vi "RangeCheck.vi"(0 "ChromaAcLoad in":refnum<class "ChromaAcLoad.lvclass">, 1 "RangeCheck":T1, 2 "Phase":i32, 3 "error in (no error)":errorcluster) -> (7 "ChromaAcLoad out":refnum<class "ChromaAcLoad.lvclass">, 10 "error out":errorcluster)   [LabVIEW 2018, in "AcPwrPlugins.lvlib" / "ChromaAcLoad.lvclass"]
doc: "This VI checks the value of the instrument settings and returns an error if the value is outside the instrument range."
uses:
  ChromaAcLoad.lvclass
  TypeDefs/RangeCheck.ctl
  <vilib>/Utility/error.llb/Error Cluster From Error Code.vi
  <vilib>/ErrorRing/Error Ring.xnode
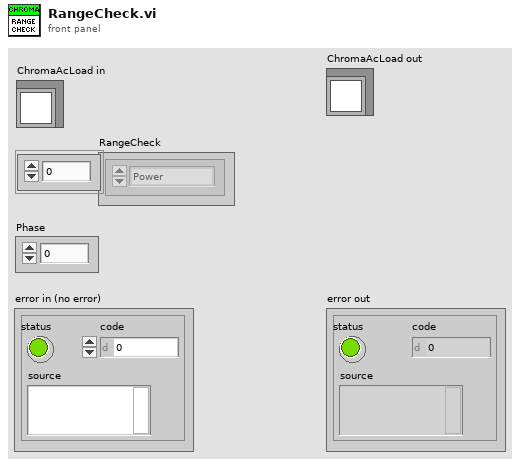
[diagram p1: front panel]
types:
  T1 = typedef "AcPwrPlugins.lvlib/ChromaAcLoad.lvclass/RangeCheck.ctl" = enum16{"Power", "AC Peak Current", "Crest Factor", "Power Factor", "Current Limit", "Current", "RLC Power Factor", "DC Peak Current", "Inrush Peak Current", "RLC Power", "DC Voltage", "AC Voltage", "DC Resistance", "AC Resistance", "Capacitance", "Inductance", "RLC RL", "RLC RS", "Frequency", "Rise Slew Rate", "Fall Slew Rate"}[]
  T2 = typedef "AcPwrPlugins.lvlib/ChromaAcLoad.lvclass/DeviceProperties.ctl" = cluster{"Frequency (Hz)":dbl, "Phases":cluster{"Handle":string, "Name":string, "Phase Select":i32, "option string ":string, "id query (Yes)":bool, "reset device (Yes)":bool, "LC":cluster{"C (uF)":i32, "L (uH)":i32, "RS (Ohm)":dbl, "RL (Ohm)":dbl}, "Load Current (A/Arms)":dbl, "Load Voltage (V/Vrms)":dbl, "Load Power (W)":dbl, "Load Resistance (Ohms)":dbl, "Load Current Peak (A)":dbl, "Load Current Limit (A/Arms)":dbl, "Slew Rate":cluster{"Rise Slew Rate (Units/S)":i32, "Fall Slew Rate (Units/S)":i32}, "Load Short Circuited":bool, "Line Synchronization":bool, "Priority":enum16{"CF Only", "PF Only", "Both (CF)", "Both (PF)"}, "Crest Factor":dbl, "Power Factor":dbl, "Connected":bool, "Voltage Range (V)":dbl[], "Timing":cluster{"TimingOn":enum16{""}, "Hours":u32, "Minutes":u32, "Seconds":dbl, "CutoffVoltage":dbl}}[], "Configuration Mode":enum16{"Constant Voltage (DC)", "Constant Power (DC)", "Constant Power (AC)", "Constant Current (DC)", "Constant Current (AC)", "Constant Resistance (DC)", "Constant Resistance (AC)", "Rectified Mode (DC)", "Inrush (AC)", "RLC CP (AC)", "RLC (AC)"}}[]
  T3 = cluster{"Handle":string, "Name":string, "Phase Select":i32, "option string ":string, "id query (Yes)":bool, "reset device (Yes)":bool, "LC":cluster{"C (uF)":i32, "L (uH)":i32, "RS (Ohm)":dbl, "RL (Ohm)":dbl}, "Load Current (A/Arms)":dbl, "Load Voltage (V/Vrms)":dbl, "Load Power (W)":dbl, "Load Resistance (Ohms)":dbl, "Load Current Peak (A)":dbl, "Load Current Limit (A/Arms)":dbl, "Slew Rate":cluster{"Rise Slew Rate (Units/S)":i32, "Fall Slew Rate (Units/S)":i32}, "Load Short Circuited":bool, "Line Synchronization":bool, "Priority":enum16{"CF Only", "PF Only", "Both (CF)", "Both (PF)"}, "Crest Factor":dbl, "Power Factor":dbl, "Connected":bool, "Voltage Range (V)":dbl[], "Timing":cluster{"TimingOn":enum16{""}, "Hours":u32, "Minutes":u32, "Seconds":dbl, "CutoffVoltage":dbl}}[]
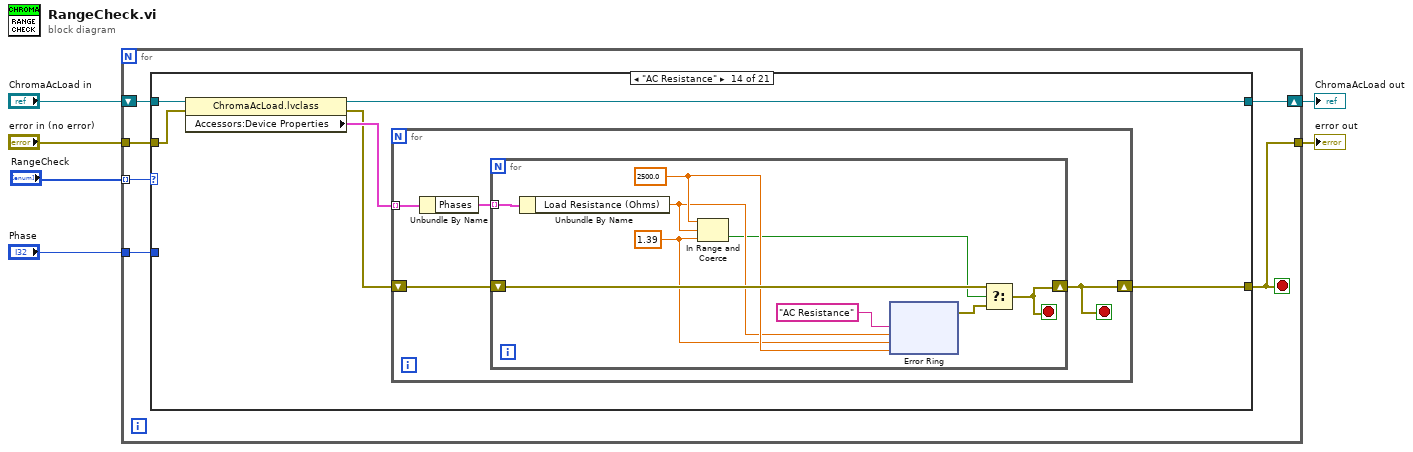
[diagram p0: block diagram]
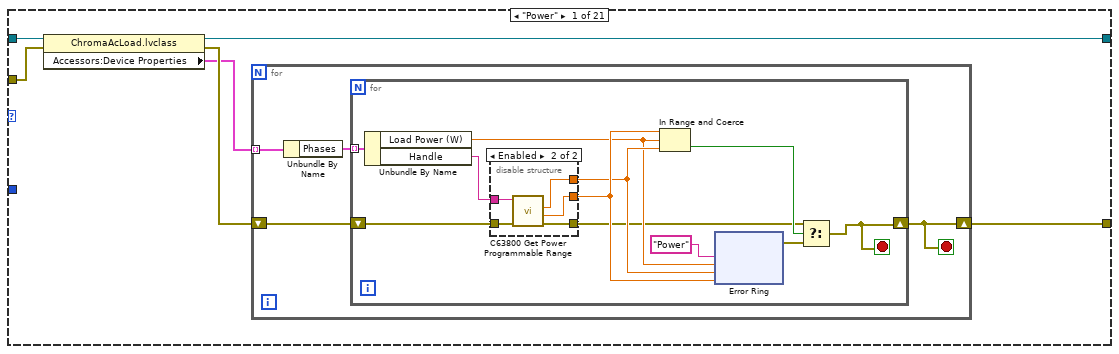
[diagram p2: hidden frame]
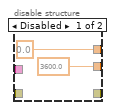
[diagram p3: hidden frame]
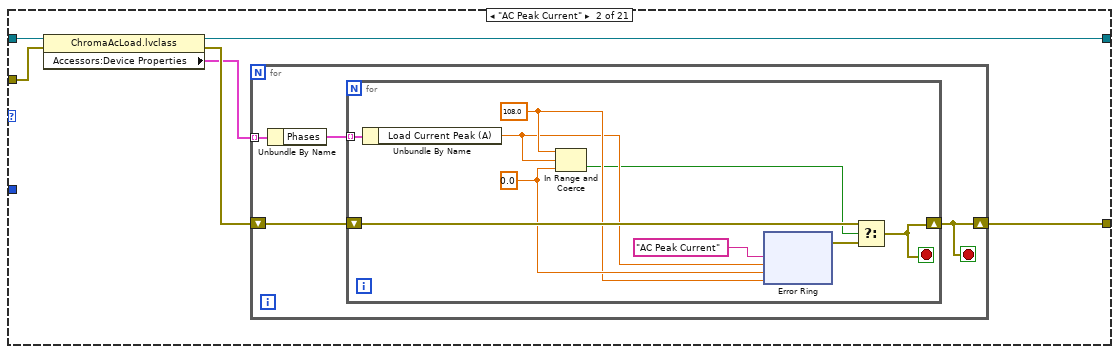
[diagram p4: hidden frame]
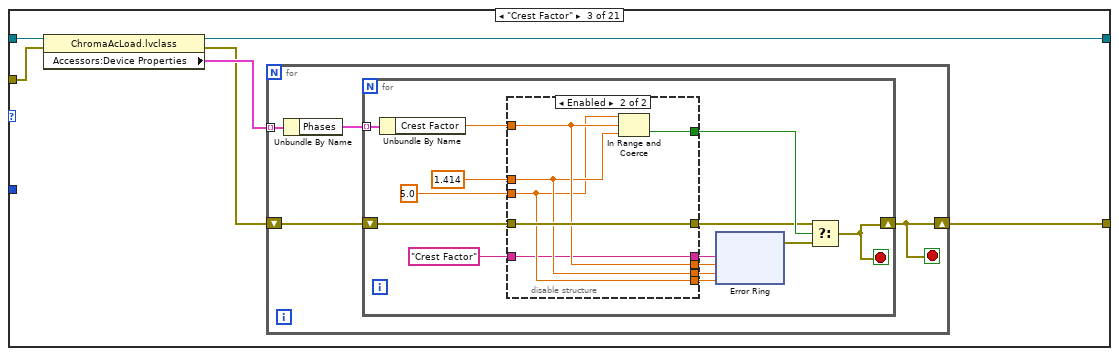
[diagram p5: hidden frame]
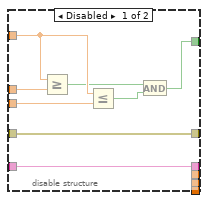
[diagram p6: hidden frame]
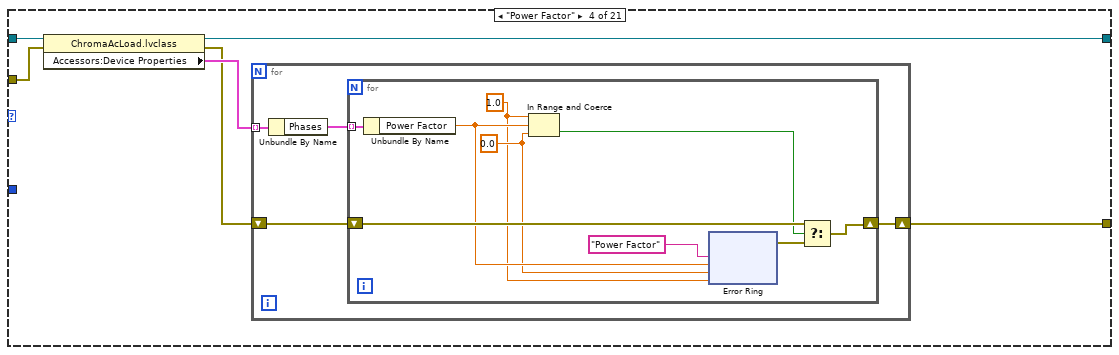
[diagram p7: hidden frame]
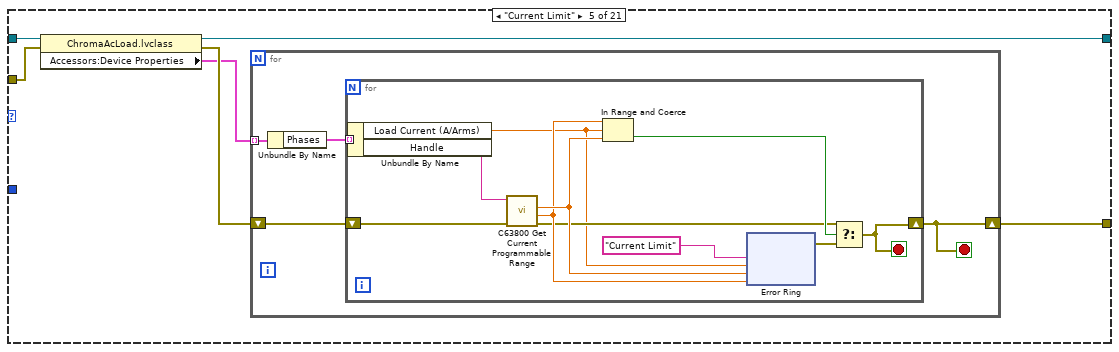
[diagram p8: hidden frame]
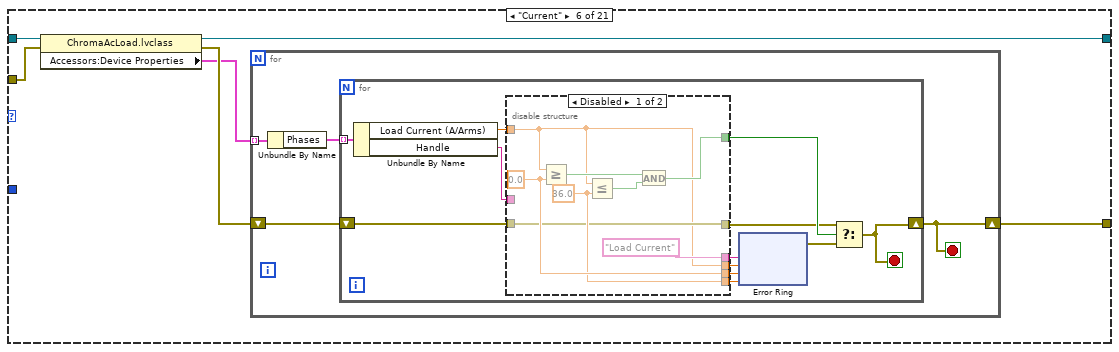
[diagram p9: hidden frame]
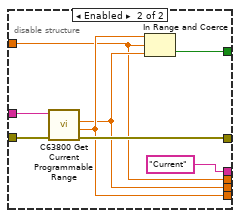
[diagram p10: hidden frame]
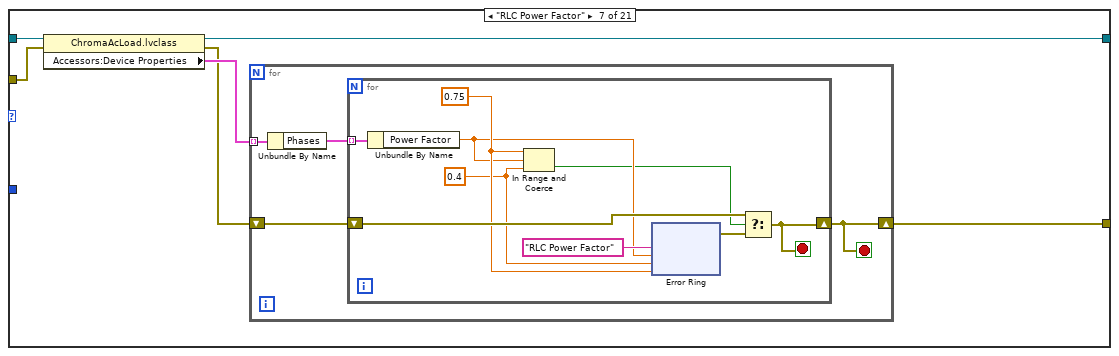
[diagram p11: hidden frame]
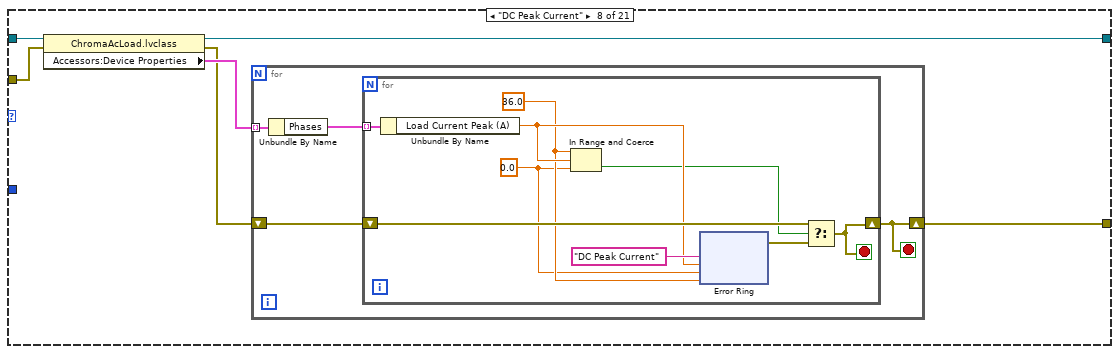
[diagram p12: hidden frame]
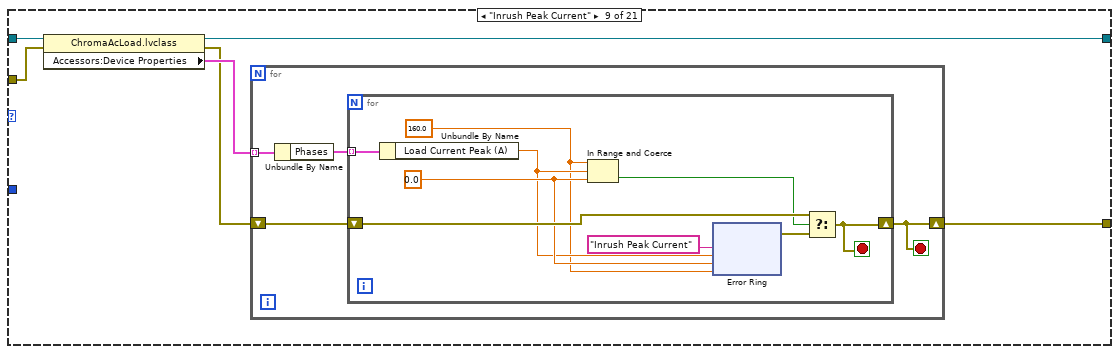
[diagram p13: hidden frame]
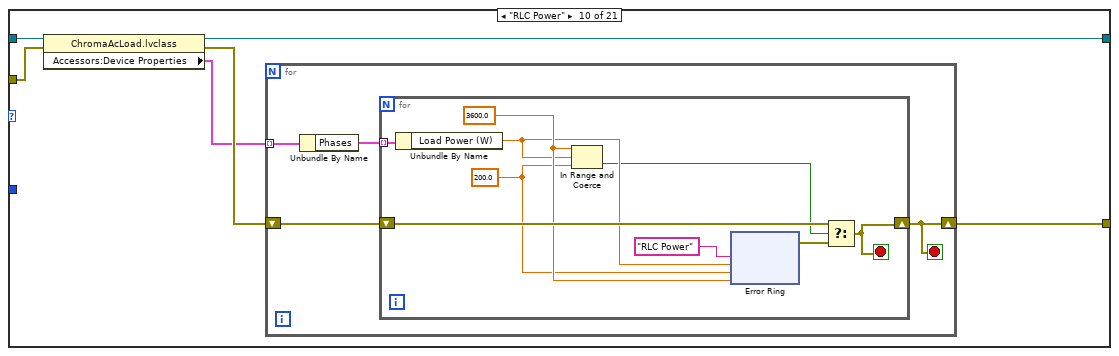
[diagram p14: hidden frame]
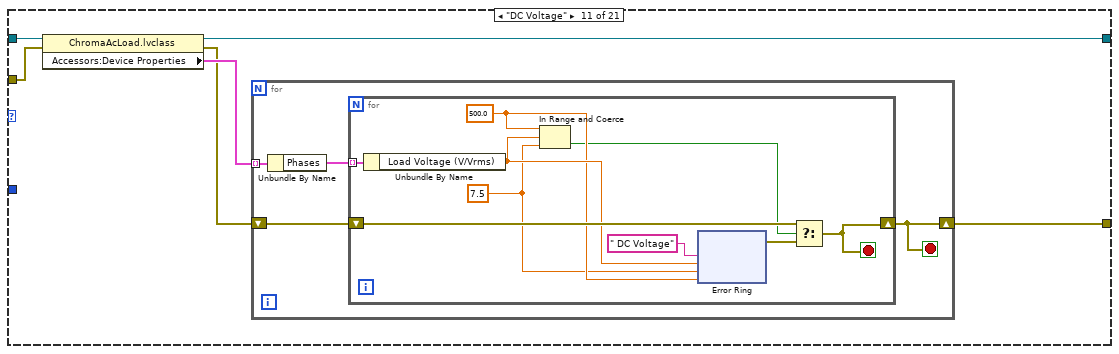
[diagram p15: hidden frame]
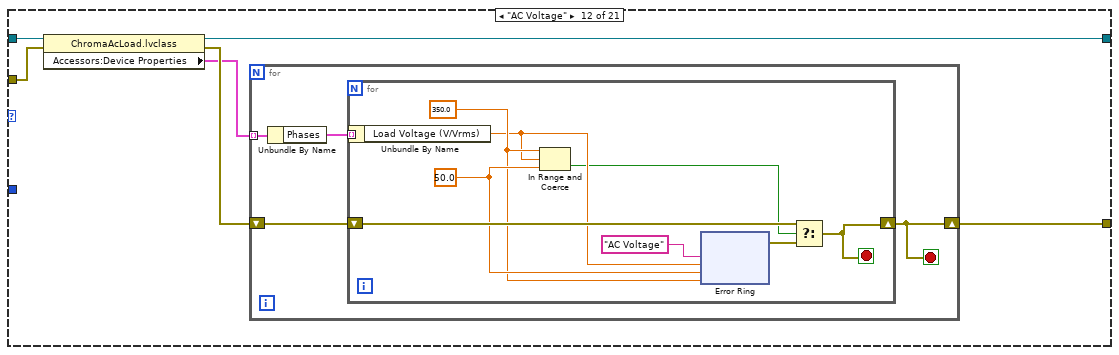
[diagram p16: hidden frame]
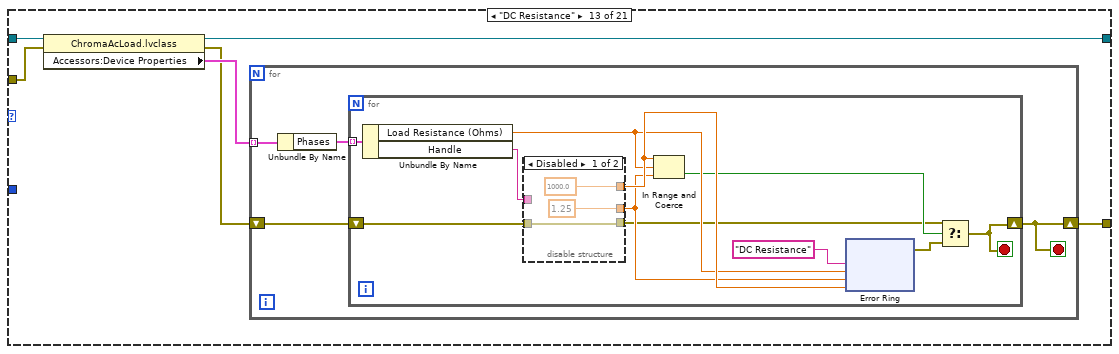
[diagram p17: hidden frame]
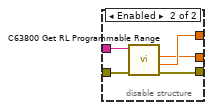
[diagram p18: hidden frame]
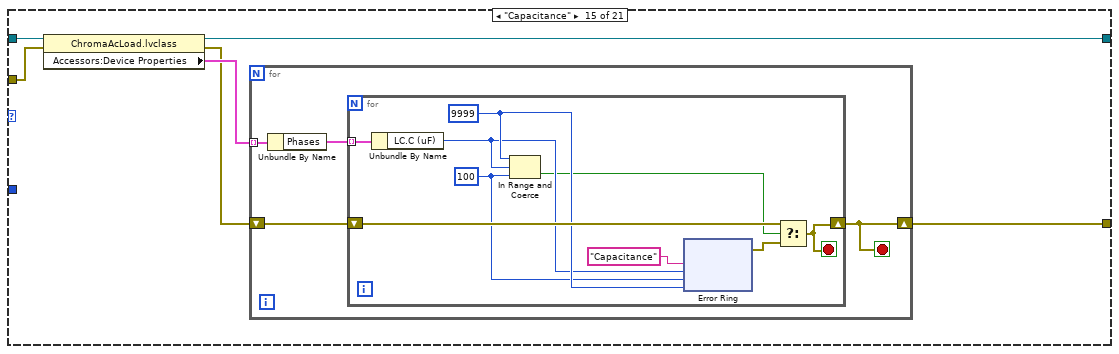
[diagram p19: hidden frame]
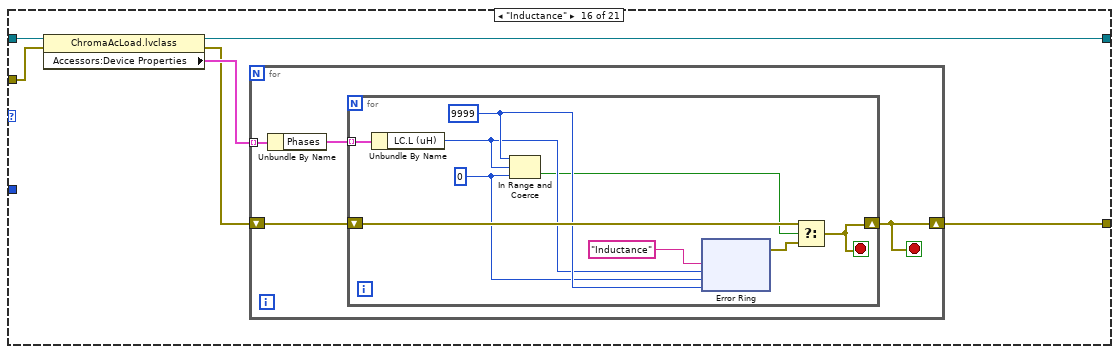
[diagram p20: hidden frame]
diagram:
  n1 = for {
    tunnel: "Phase" -> [w11]
    shift-right: [w10] -> w4
    shift-left: "ChromaAcLoad in" -> [w12]
    tunnel: [w9] -> w3
    tunnel: "error in (no error)" -> [w8]
    tunnel: "RangeCheck" -> [w7] mode=indexing
    stop <- w9 stop-if-true
    n2 = case shown="\"AC Resistance\"" w7 {
      tunnel: w12 -> [w18 w56 w85 w133 w162 w193 w241 w270 w299 w328 w357 w386 w415 w454 w483 w512 w541 w570 w599 w624 w653]
      tunnel: w11 -> [_ _ _ _ _ _ _ _ _ _ _ _ _ _ _ _ _ _ _ _ _]
      tunnel: [w17 w55 w83 w131 w161 w192 w239 w268 w297 w327 w355 w385 w413 w452 w481 w510 w539 w568 w597 w622 w651] -> w10
      tunnel: [w15 w53 w81 w129 w159 w190 w237 w266 w295 w325 w353 w383 w411 w450 w479 w508 w537 w566 w595 w620 w649] -> w9
      tunnel: w8 -> [w14 w52 w80 w128 w158 w189 w236 w265 w294 w324 w352 w382 w410 w449 w478 w507 w536 w565 w594 w619 w648]
      frame "Power" {
        n3 = property class="ChromaAcLoad.lvclass"(reference=w18, error in=w14) -> (reference out=w17:refnum<class "ChromaAcLoad.lvclass">, error out=w16:errorcluster, "Accessors:Device Properties"=w13:T2)
        n4 = for {
          shift-right: [w19] -> w15
          shift-left: w16 -> [w22]
          tunnel: w13 -> [w21] mode=indexing
          stop <- w19 stop-if-true
          n5 = Unbundle By Name(w21) -> ("Phases"=w20:T3)
          n6 = for {
            shift-right: [w27] -> w19
            shift-left: w22 -> [w25]
            tunnel: w20 -> [w31] mode=indexing
            stop <- w27 stop-if-true
            n7 = Unbundle By Name(w31) -> ("Load Power (W)"=w26:dbl, "Handle"=w23:string)
            n8 = disable-structure shown="Enabled" {
              disable-tunnel: [3600.0 w38] -> w30
              disable-tunnel: [0.0 w37] -> w29
              disable-tunnel: w25 -> [_ w40]
              disable-tunnel: [_ w39] -> w24
              disable-tunnel: w23 -> [_ w36]
              frame Disabled {
              }
              frame Enabled {
                n9 = call <instrlib>:"C63800 Get Power Programmable Range.vi"("error in (no error)"=w40, "Instrument Handle"=w36) -> ("error out"=w39:errorcluster, "Maximum"=w38:dbl, "Minimum"=w37:dbl)  [unwired: 6 in, 1 out]
              }
            }
            n10 = In Range and Coerce(upper limit=w30, x=w26, lower limit=w29) -> (In Range?=w28:bool)  [unwired: 1 out]
            n11 = xnode "Error Ring"("parameter 0"="Power", "parameter 1"=w26, "parameter 2"=w29, "parameter 3"=w30) -> ("error out"=w32:errorcluster)
            n12 = Select(t=w24, s=w28, f=w32) -> (s? t:f=w27:errorcluster)
          }
        }
      }
      frame "AC Peak Current" {
        n13 = property class="ChromaAcLoad.lvclass"(reference=w56, error in=w52) -> (reference out=w55:refnum<class "ChromaAcLoad.lvclass">, error out=w54:errorcluster, "Accessors:Device Properties"=w51:T2)
        n14 = for {
          tunnel: w51 -> [w59] mode=indexing
          shift-right: [w57] -> w53
          shift-left: w54 -> [w60]
          stop <- w57 stop-if-true
          n15 = Unbundle By Name(w59) -> ("Phases"=w58:T3)
          n16 = for {
            shift-right: [w61] -> w57
            shift-left: w60 -> [w67]
            tunnel: w58 -> [w66] mode=indexing
            stop <- w61 stop-if-true
            w65 = 0.0
            w64 = 108.0
            n17 = Unbundle By Name(w66) -> ("Load Current Peak (A)"=w63:dbl)
            n18 = In Range and Coerce(upper limit=w64, x=w63, lower limit=w65) -> (In Range?=w62:bool)  [unwired: 1 out]
            n19 = xnode "Error Ring"("parameter 0"="AC Peak Current", "parameter 1"=w63, "parameter 2"=w65, "parameter 3"=w64) -> ("error out"=w68:errorcluster)
            n20 = Select(t=w67, s=w62, f=w68) -> (s? t:f=w61:errorcluster)
          }
        }
      }
      frame "Crest Factor" {
        n21 = property class="ChromaAcLoad.lvclass"(reference=w85, error in=w80) -> (reference out=w83:refnum<class "ChromaAcLoad.lvclass">, error out=w82:errorcluster, "Accessors:Device Properties"=w84:T2)
        n22 = for {
          tunnel: w84 -> [w88] mode=indexing
          shift-right: [w86] -> w81
          shift-left: w82 -> [w89]
          stop <- w86 stop-if-true
          n23 = Unbundle By Name(w88) -> ("Phases"=w87:T3)
          n24 = for {
            shift-right: [w90] -> w86
            shift-left: w89 -> [w97]
            tunnel: w87 -> [w98] mode=indexing
            stop <- w90 stop-if-true
            n25 = Unbundle By Name(w98) -> ("Crest Factor"=w103:dbl)
            n26 = disable-structure shown="Enabled" {
              disable-tunnel: w103 -> [w111 w115]
              disable-tunnel: [w108 w116] -> w102
              disable-tunnel: 1.414 -> [w107 w114]
              disable-tunnel: 5.0 -> [w106 w113]
              disable-tunnel: w97 -> [w104 w117]
              disable-tunnel: [w104 w117] -> w96
              disable-tunnel: [_ w115] -> w95
              disable-tunnel: [_ w114] -> w94
              disable-tunnel: [_ w113] -> w93
              disable-tunnel: "Crest Factor" -> [w105 w112]
              disable-tunnel: [w105 w112] -> w91
              frame Disabled {
                n27 = Greater Or Equal?(x=w111, y=w107) -> (x >= y?=w110:bool)
                n28 = Less Or Equal?(x=w111, y=w106) -> (x <= y?=w109:bool)
                n29 = And(x=w110, y=w109) -> (x .and. y?=w108:bool)
              }
              frame Enabled {
                n30 = In Range and Coerce(upper limit=w113, x=w115, lower limit=w114) -> (In Range?=w116:bool)  [unwired: 1 out]
              }
            }
            n31 = xnode "Error Ring"("parameter 0"=w91, "parameter 1"=w95, "parameter 2"=w94, "parameter 3"=w93) -> ("error out"=w101:errorcluster)
            n32 = Select(t=w96, s=w102, f=w101) -> (s? t:f=w90:errorcluster)
          }
        }
      }
      frame "Power Factor" {
        n33 = property class="ChromaAcLoad.lvclass"(reference=w133, error in=w128) -> (reference out=w131:refnum<class "ChromaAcLoad.lvclass">, error out=w130:errorcluster, "Accessors:Device Properties"=w132:T2)
        n34 = for {
          tunnel: w132 -> [w135] mode=indexing
          shift-right: [w136] -> w129
          shift-left: w130 -> [w137]
          n35 = Unbundle By Name(w135) -> ("Phases"=w134:T3)
          n36 = for {
            shift-right: [w143] -> w136
            shift-left: w137 -> [w144]
            tunnel: w134 -> [w142] mode=indexing
            w139 = 1.0
            w140 = 0.0
            n37 = Unbundle By Name(w142) -> ("Power Factor"=w141:dbl)
            n38 = In Range and Coerce(upper limit=w139, x=w141, lower limit=w140) -> (In Range?=w138:bool)  [unwired: 1 out]
            n39 = xnode "Error Ring"("parameter 0"="Power Factor", "parameter 1"=w141, "parameter 2"=w140, "parameter 3"=w139) -> ("error out"=w145:errorcluster)
            n40 = Select(t=w144, s=w138, f=w145) -> (s? t:f=w143:errorcluster)
          }
        }
      }
      frame "Current Limit" {
        n41 = property class="ChromaAcLoad.lvclass"(reference=w162, error in=w158) -> (reference out=w161:refnum<class "ChromaAcLoad.lvclass">, error out=w160:errorcluster, "Accessors:Device Properties"=w157:T2)
        n42 = for {
          tunnel: w157 -> [w166] mode=indexing
          shift-right: [w163] -> w159
          shift-left: w160 -> [w164]
          stop <- w163 stop-if-true
          n43 = Unbundle By Name(w166) -> ("Phases"=w165:T3)
          n44 = for {
            tunnel: w165 -> [w172] mode=indexing
            shift-right: [w167] -> w163
            shift-left: w164 -> [w171]
            stop <- w167 stop-if-true
            n45 = Unbundle By Name(w172) -> ("Load Current (A/Arms)"=w168:dbl, "Handle"=w169:string)
            n46 = call <instrlib>:"C63800 Get Current Programmable Range.vi"("error in (no error)"=w171, "Instrument Handle"=w169) -> ("error out"=w170:errorcluster, "Maximum"=w173:dbl, "Minimum"=w174:dbl)  [unwired: 6 in, 1 out]
            n47 = In Range and Coerce(upper limit=w173, x=w168, lower limit=w174) -> (In Range?=w176:bool)  [unwired: 1 out]
            n48 = xnode "Error Ring"("parameter 0"="Current Limit", "parameter 1"=w168, "parameter 2"=w174, "parameter 3"=w173) -> ("error out"=w175:errorcluster)
            n49 = Select(t=w170, s=w176, f=w175) -> (s? t:f=w167:errorcluster)
          }
        }
      }
      frame "Current" {
        n50 = property class="ChromaAcLoad.lvclass"(reference=w193, error in=w189) -> (reference out=w192:refnum<class "ChromaAcLoad.lvclass">, error out=w191:errorcluster, "Accessors:Device Properties"=w188:T2)
        n51 = for {
          tunnel: w188 -> [w197] mode=indexing
          shift-right: [w194] -> w190
          shift-left: w191 -> [w195]
          stop <- w194 stop-if-true
          n52 = Unbundle By Name(w197) -> ("Phases"=w196:T3)
          n53 = for {
            tunnel: w196 -> [w204] mode=indexing
            shift-right: [w198] -> w194
            shift-left: w195 -> [w202]
            stop <- w198 stop-if-true
            n54 = Unbundle By Name(w204) -> ("Load Current (A/Arms)"=w203:dbl, "Handle"=w200:string)
            n55 = disable-structure shown="Disabled" {
              disable-tunnel: ["Load Current" "Current"] -> w209
              disable-tunnel: [w214 w222] -> w208
              disable-tunnel: [w213 w220] -> w206
              disable-tunnel: [w212 w221] -> w205
              disable-tunnel: w203 -> [w210 w219]
              disable-tunnel: w202 -> [w211 w225]
              disable-tunnel: [w211 w224] -> w201
              disable-tunnel: w200 -> [_ w223]
              disable-tunnel: [w210 w219] -> w199
              frame Disabled {
                w212 = 36.0
                w213 = 0.0
                n56 = Greater Or Equal?(x=w210, y=w213) -> (x >= y?=w216:bool)
                n57 = Less Or Equal?(x=w210, y=w212) -> (x <= y?=w215:bool)
                n58 = And(x=w216, y=w215) -> (x .and. y?=w214:bool)
              }
              frame Enabled {
                n59 = call <instrlib>:"C63800 Get Current Programmable Range.vi"("error in (no error)"=w225, "Instrument Handle"=w223) -> ("error out"=w224:errorcluster, "Maximum"=w221:dbl, "Minimum"=w220:dbl)  [unwired: 6 in, 1 out]
                n60 = In Range and Coerce(upper limit=w221, x=w219, lower limit=w220) -> (In Range?=w222:bool)  [unwired: 1 out]
              }
            }
            n61 = xnode "Error Ring"("parameter 0"=w209, "parameter 1"=w199, "parameter 2"=w206, "parameter 3"=w205) -> ("error out"=w207:errorcluster)
            n62 = Select(t=w201, s=w208, f=w207) -> (s? t:f=w198:errorcluster)
          }
        }
      }
      frame "RLC Power Factor" {
        n63 = property class="ChromaAcLoad.lvclass"(reference=w241, error in=w236) -> (reference out=w239:refnum<class "ChromaAcLoad.lvclass">, error out=w238:errorcluster, "Accessors:Device Properties"=w240:T2)
        n64 = for {
          tunnel: w240 -> [w244] mode=indexing
          shift-right: [w242] -> w237
          shift-left: w238 -> [w245]
          stop <- w242 stop-if-true
          n65 = Unbundle By Name(w244) -> ("Phases"=w243:T3)
          n66 = for {
            tunnel: w243 -> [w248] mode=indexing
            shift-right: [w247] -> w242
            shift-left: w245 -> [w252]
            stop <- w247 stop-if-true
            w251 = 0.75
            w249 = 0.4
            n67 = Unbundle By Name(w248) -> ("Power Factor"=w250:dbl)
            n68 = In Range and Coerce(upper limit=w251, x=w250, lower limit=w249) -> (In Range?=w246:bool)  [unwired: 1 out]
            n69 = xnode "Error Ring"("parameter 0"="RLC Power Factor", "parameter 1"=w250, "parameter 2"=w249, "parameter 3"=w251) -> ("error out"=w253:errorcluster)
            n70 = Select(t=w252, s=w246, f=w253) -> (s? t:f=w247:errorcluster)
          }
        }
      }
      frame "DC Peak Current" {
        n71 = property class="ChromaAcLoad.lvclass"(reference=w270, error in=w265) -> (reference out=w268:refnum<class "ChromaAcLoad.lvclass">, error out=w267:errorcluster, "Accessors:Device Properties"=w269:T2)
        n72 = for {
          tunnel: w269 -> [w273] mode=indexing
          shift-right: [w271] -> w266
          shift-left: w267 -> [w274]
          stop <- w271 stop-if-true
          n73 = Unbundle By Name(w273) -> ("Phases"=w272:T3)
          n74 = for {
            shift-right: [w275] -> w271
            shift-left: w274 -> [w281]
            tunnel: w272 -> [w280] mode=indexing
            stop <- w275 stop-if-true
            w278 = 36.0
            w277 = 0.0
            n75 = Unbundle By Name(w280) -> ("Load Current Peak (A)"=w279:dbl)
            n76 = In Range and Coerce(upper limit=w278, x=w279, lower limit=w277) -> (In Range?=w276:bool)  [unwired: 1 out]
            n77 = xnode "Error Ring"("parameter 0"="DC Peak Current", "parameter 1"=w279, "parameter 2"=w277, "parameter 3"=w278) -> ("error out"=w282:errorcluster)
            n78 = Select(t=w281, s=w276, f=w282) -> (s? t:f=w275:errorcluster)
          }
        }
      }
      frame "Inrush Peak Current" {
        n79 = property class="ChromaAcLoad.lvclass"(reference=w299, error in=w294) -> (reference out=w297:refnum<class "ChromaAcLoad.lvclass">, error out=w296:errorcluster, "Accessors:Device Properties"=w298:T2)
        n80 = for {
          tunnel: w298 -> [w302] mode=indexing
          shift-right: [w300] -> w295
          shift-left: w296 -> [w303]
          stop <- w300 stop-if-true
          n81 = Unbundle By Name(w302) -> ("Phases"=w301:T3)
          n82 = for {
            shift-right: [w308] -> w300
            shift-left: w303 -> [w310]
            tunnel: w301 -> [w309] mode=indexing
            stop <- w308 stop-if-true
            w305 = 160.0
            w307 = 0.0
            n83 = Unbundle By Name(w309) -> ("Load Current Peak (A)"=w306:dbl)
            n84 = In Range and Coerce(upper limit=w305, x=w306, lower limit=w307) -> (In Range?=w304:bool)  [unwired: 1 out]
            n85 = xnode "Error Ring"("parameter 0"="Inrush Peak Current", "parameter 1"=w306, "parameter 2"=w307, "parameter 3"=w305) -> ("error out"=w311:errorcluster)
            n86 = Select(t=w310, s=w304, f=w311) -> (s? t:f=w308:errorcluster)
          }
        }
      }
      frame "RLC Power" {
        n87 = property class="ChromaAcLoad.lvclass"(reference=w328, error in=w324) -> (reference out=w327:refnum<class "ChromaAcLoad.lvclass">, error out=w326:errorcluster, "Accessors:Device Properties"=w323:T2)
        n88 = for {
          shift-right: [w329] -> w325
          shift-left: w326 -> [w332]
          tunnel: w323 -> [w331] mode=indexing
          stop <- w329 stop-if-true
          n89 = Unbundle By Name(w331) -> ("Phases"=w330:T3)
          n90 = for {
            shift-right: [w337] -> w329
            shift-left: w332 -> [w339]
            tunnel: w330 -> [w338] mode=indexing
            stop <- w337 stop-if-true
            w336 = 3600.0
            w335 = 200.0
            n91 = Unbundle By Name(w338) -> ("Load Power (W)"=w334:dbl)
            n92 = In Range and Coerce(upper limit=w336, x=w334, lower limit=w335) -> (In Range?=w333:bool)  [unwired: 1 out]
            n93 = xnode "Error Ring"("parameter 0"="RLC Power", "parameter 1"=w334, "parameter 2"=w335, "parameter 3"=w336) -> ("error out"=w340:errorcluster)
            n94 = Select(t=w339, s=w333, f=w340) -> (s? t:f=w337:errorcluster)
          }
        }
      }
      frame "DC Voltage" {
        n95 = property class="ChromaAcLoad.lvclass"(reference=w357, error in=w352) -> (reference out=w355:refnum<class "ChromaAcLoad.lvclass">, error out=w354:errorcluster, "Accessors:Device Properties"=w356:T2)
        n96 = for {
          tunnel: w356 -> [w359] mode=indexing
          shift-right: [w360] -> w353
          shift-left: w354 -> [w361]
          stop <- w360 stop-if-true
          n97 = Unbundle By Name(w359) -> ("Phases"=w358:T3)
          n98 = for {
            shift-right: [w367] -> w360
            shift-left: w361 -> [w368]
            tunnel: w358 -> [w366] mode=indexing
            stop <- w367 stop-if-true
            w364 = 500.0
            w363 = 7.5
            n99 = Unbundle By Name(w366) -> ("Load Voltage (V/Vrms)"=w365:dbl)
            n100 = In Range and Coerce(upper limit=w364, x=w365, lower limit=w363) -> (In Range?=w362:bool)  [unwired: 1 out]
            n101 = xnode "Error Ring"("parameter 0"=" DC Voltage", "parameter 1"=w365, "parameter 2"=w363, "parameter 3"=w364) -> ("error out"=w369:errorcluster)
            n102 = Select(t=w368, s=w362, f=w369) -> (s? t:f=w367:errorcluster)
          }
        }
      }
      frame "AC Voltage" {
        n103 = property class="ChromaAcLoad.lvclass"(reference=w386, error in=w382) -> (reference out=w385:refnum<class "ChromaAcLoad.lvclass">, error out=w384:errorcluster, "Accessors:Device Properties"=w381:T2)
        n104 = for {
          shift-right: [w387] -> w383
          shift-left: w384 -> [w390]
          tunnel: w381 -> [w389] mode=indexing
          stop <- w387 stop-if-true
          n105 = Unbundle By Name(w389) -> ("Phases"=w388:T3)
          n106 = for {
            shift-right: [w391] -> w387
            shift-left: w390 -> [w397]
            tunnel: w388 -> [w396] mode=indexing
            stop <- w391 stop-if-true
            w394 = 350.0
            w395 = 50.0
            n107 = Unbundle By Name(w396) -> ("Load Voltage (V/Vrms)"=w393:dbl)
            n108 = In Range and Coerce(upper limit=w394, x=w393, lower limit=w395) -> (In Range?=w392:bool)  [unwired: 1 out]
            n109 = xnode "Error Ring"("parameter 0"="AC Voltage", "parameter 1"=w393, "parameter 2"=w395, "parameter 3"=w394) -> ("error out"=w398:errorcluster)
            n110 = Select(t=w397, s=w392, f=w398) -> (s? t:f=w391:errorcluster)
          }
        }
      }
      frame "DC Resistance" {
        n111 = property class="ChromaAcLoad.lvclass"(reference=w415, error in=w410) -> (reference out=w413:refnum<class "ChromaAcLoad.lvclass">, error out=w412:errorcluster, "Accessors:Device Properties"=w414:T2)
        n112 = for {
          tunnel: w414 -> [w417] mode=indexing
          shift-right: [w418] -> w411
          shift-left: w412 -> [w419]
          stop <- w418 stop-if-true
          n113 = Unbundle By Name(w417) -> ("Phases"=w416:T3)
          n114 = for {
            shift-right: [w428] -> w418
            shift-left: w419 -> [w422]
            tunnel: w416 -> [w427] mode=indexing
            stop <- w428 stop-if-true
            n115 = Unbundle By Name(w427) -> ("Load Resistance (Ohms)"=w425:dbl, "Handle"=w420:string)
            n116 = disable-structure shown="Disabled" {
              disable-tunnel: [1000.0 w436] -> w426
              disable-tunnel: [1.25 w435] -> w423
              disable-tunnel: w422 -> [w431 w438]
              disable-tunnel: [w431 w437] -> w421
              disable-tunnel: w420 -> [_ w434]
              frame Disabled {
              }
              frame Enabled {
                n117 = call <instrlib>:"C63800 Get RL Programmable Range.vi"("error in (no error)"=w438, "Instrument Handle"=w434) -> ("error out"=w437:errorcluster, "Maximum"=w436:dbl, "Minimum"=w435:dbl)  [unwired: 6 in, 1 out]
              }
            }
            n118 = In Range and Coerce(upper limit=w426, x=w425, lower limit=w423) -> (In Range?=w424:bool)  [unwired: 1 out]
            n119 = xnode "Error Ring"("parameter 0"="DC Resistance", "parameter 1"=w425, "parameter 2"=w423, "parameter 3"=w426) -> ("error out"=w429:errorcluster)
            n120 = Select(t=w421, s=w424, f=w429) -> (s? t:f=w428:errorcluster)
          }
        }
      }
      frame "AC Resistance" {
        n121 = property class="ChromaAcLoad.lvclass"(reference=w454, error in=w449) -> (reference out=w452:refnum<class "ChromaAcLoad.lvclass">, error out=w451:errorcluster, "Accessors:Device Properties"=w453:T2)
        n122 = for {
          tunnel: w453 -> [w456] mode=indexing
          shift-right: [w457] -> w450
          shift-left: w451 -> [w458]
          stop <- w457 stop-if-true
          n123 = Unbundle By Name(w456) -> ("Phases"=w455:T3)
          n124 = for {
            shift-right: [w464] -> w457
            shift-left: w458 -> [w465]
            tunnel: w455 -> [w463] mode=indexing
            stop <- w464 stop-if-true
            w462 = 2500.0
            w459 = 1.39
            n125 = Unbundle By Name(w463) -> ("Load Resistance (Ohms)"=w461:dbl)
            n126 = In Range and Coerce(upper limit=w462, x=w461, lower limit=w459) -> (In Range?=w460:bool)  [unwired: 1 out]
            n127 = xnode "Error Ring"("parameter 0"="AC Resistance", "parameter 1"=w461, "parameter 2"=w459, "parameter 3"=w462) -> ("error out"=w466:errorcluster)
            n128 = Select(t=w465, s=w460, f=w466) -> (s? t:f=w464:errorcluster)
          }
        }
      }
      frame "Capacitance" {
        n129 = property class="ChromaAcLoad.lvclass"(reference=w483, error in=w478) -> (reference out=w481:refnum<class "ChromaAcLoad.lvclass">, error out=w480:errorcluster, "Accessors:Device Properties"=w482:T2)
        n130 = for {
          tunnel: w482 -> [w485] mode=indexing
          shift-right: [w486] -> w479
          shift-left: w480 -> [w487]
          stop <- w486 stop-if-true
          n131 = Unbundle By Name(w485) -> ("Phases"=w484:T3)
          n132 = for {
            shift-right: [w493] -> w486
            shift-left: w487 -> [w494]
            tunnel: w484 -> [w492] mode=indexing
            stop <- w493 stop-if-true
            w491 = 9999
            w488 = 100
            n133 = Unbundle By Name(w492) -> ("LC.C (uF)"=w490:i32)
            n134 = In Range and Coerce(upper limit=w491, x=w490, lower limit=w488) -> (In Range?=w489:bool)  [unwired: 1 out]
            n135 = xnode "Error Ring"("parameter 0"="Capacitance", "parameter 1"=w490, "parameter 2"=w488, "parameter 3"=w491) -> ("error out"=w495:errorcluster)
            n136 = Select(t=w494, s=w489, f=w495) -> (s? t:f=w493:errorcluster)
          }
        }
      }
      frame "Inductance" {
        n137 = property class="ChromaAcLoad.lvclass"(reference=w512, error in=w507) -> (reference out=w510:refnum<class "ChromaAcLoad.lvclass">, error out=w509:errorcluster, "Accessors:Device Properties"=w511:T2)
        n138 = for {
          tunnel: w511 -> [w514] mode=indexing
          shift-right: [w515] -> w508
          shift-left: w509 -> [w516]
          stop <- w515 stop-if-true
          n139 = Unbundle By Name(w514) -> ("Phases"=w513:T3)
          n140 = for {
            shift-right: [w522] -> w515
            shift-left: w516 -> [w523]
            tunnel: w513 -> [w521] mode=indexing
            stop <- w522 stop-if-true
            w520 = 9999
            w517 = 0
            n141 = Unbundle By Name(w521) -> ("LC.L (uH)"=w519:i32)
            n142 = In Range and Coerce(upper limit=w520, x=w519, lower limit=w517) -> (In Range?=w518:bool)  [unwired: 1 out]
            n143 = xnode "Error Ring"("parameter 0"="Inductance", "parameter 1"=w519, "parameter 2"=w517, "parameter 3"=w520) -> ("error out"=w524:errorcluster)
            n144 = Select(t=w523, s=w518, f=w524) -> (s? t:f=w522:errorcluster)
          }
        }
      }
      frame "RLC RL" {
        n145 = property class="ChromaAcLoad.lvclass"(reference=w541, error in=w536) -> (reference out=w539:refnum<class "ChromaAcLoad.lvclass">, error out=w538:errorcluster, "Accessors:Device Properties"=w540:T2)
        n146 = for {
          tunnel: w540 -> [w543] mode=indexing
          shift-right: [w544] -> w537
          shift-left: w538 -> [w545]
          stop <- w544 stop-if-true
          n147 = Unbundle By Name(w543) -> ("Phases"=w542:T3)
          n148 = for {
            shift-right: [w551] -> w544
            shift-left: w545 -> [w552]
            tunnel: w542 -> [w550] mode=indexing
            stop <- w551 stop-if-true
            w549 = 9999.99
            w546 = 1.39
            n149 = Unbundle By Name(w550) -> ("LC.RL (Ohm)"=w548:dbl)
            n150 = In Range and Coerce(upper limit=w549, x=w548, lower limit=w546) -> (In Range?=w547:bool)  [unwired: 1 out]
            n151 = xnode "Error Ring"("parameter 0"="Parallel Resistance", "parameter 1"=w548, "parameter 2"=w546, "parameter 3"=w549) -> ("error out"=w553:errorcluster)
            n152 = Select(t=w552, s=w547, f=w553) -> (s? t:f=w551:errorcluster)
          }
        }
      }
      frame "RLC RS" {
        n153 = property class="ChromaAcLoad.lvclass"(reference=w570, error in=w565) -> (reference out=w568:refnum<class "ChromaAcLoad.lvclass">, error out=w567:errorcluster, "Accessors:Device Properties"=w569:T2)
        n154 = for {
          tunnel: w569 -> [w572] mode=indexing
          shift-right: [w573] -> w566
          shift-left: w567 -> [w574]
          stop <- w573 stop-if-true
          n155 = Unbundle By Name(w572) -> ("Phases"=w571:T3)
          n156 = for {
            shift-right: [w580] -> w573
            shift-left: w574 -> [w581]
            tunnel: w571 -> [w579] mode=indexing
            stop <- w580 stop-if-true
            w578 = 9.999
            w575 = 1.39
            n157 = Unbundle By Name(w579) -> ("LC.RL (Ohm)"=w577:dbl)
            n158 = In Range and Coerce(upper limit=w578, x=w577, lower limit=w575) -> (In Range?=w576:bool)  [unwired: 1 out]
            n159 = xnode "Error Ring"("parameter 0"="Series Resistance", "parameter 1"=w577, "parameter 2"=w575, "parameter 3"=w578) -> ("error out"=w582:errorcluster)
            n160 = Select(t=w581, s=w576, f=w582) -> (s? t:f=w580:errorcluster)
          }
        }
      }
      frame "Frequency" {
        n161 = property class="ChromaAcLoad.lvclass"(reference=w599, error in=w594) -> (reference out=w597:refnum<class "ChromaAcLoad.lvclass">, error out=w596:errorcluster, "Accessors:Device Properties"=w598:T2)
        n162 = for {
          tunnel: w598 -> [w606] mode=indexing
          shift-right: [w607] -> w595
          shift-left: w596 -> [w608]
          stop <- w607 stop-if-true
          w603 = 440.0
          w601 = 45.0
          n163 = Unbundle By Name(w606) -> ("Frequency (Hz)"=w600:dbl)
          n164 = In Range and Coerce(upper limit=w603, x=w600, lower limit=w601) -> (In Range?=w602:bool)  [unwired: 1 out]
          n165 = xnode "Error Ring"("parameter 0"="Frequency", "parameter 1"=w600, "parameter 2"=w601, "parameter 3"=w603) -> ("error out"=w604:errorcluster)
          n166 = Select(t=w608, s=w602, f=w604) -> (s? t:f=w607:errorcluster)
        }
      }
      frame "Rise Slew Rate" {
        n167 = property class="ChromaAcLoad.lvclass"(reference=w624, error in=w619) -> (reference out=w622:refnum<class "ChromaAcLoad.lvclass">, error out=w621:errorcluster, "Accessors:Device Properties"=w623:T2)
        n168 = for {
          tunnel: w623 -> [w626] mode=indexing
          shift-right: [w627] -> w620
          shift-left: w621 -> [w628]
          stop <- w627 stop-if-true
          n169 = Unbundle By Name(w626) -> ("Phases"=w625:T3)
          n170 = for {
            shift-right: [w634] -> w627
            shift-left: w628 -> [w635]
            tunnel: w625 -> [w633] mode=indexing
            stop <- w634 stop-if-true
            w629 = 4
            w630 = 600
            n171 = Unbundle By Name(w633) -> ("Slew Rate.Rise Slew Rate (Units/S)"=w632:i32)
            n172 = In Range and Coerce(upper limit=w630, x=w632, lower limit=w629) -> (In Range?=w631:bool)  [unwired: 1 out]
            n173 = xnode "Error Ring"("parameter 0"="Rise Slew Rate", "parameter 1"=w632, "parameter 2"=w629, "parameter 3"=w630) -> ("error out"=w636:errorcluster)
            n174 = Select(t=w635, s=w631, f=w636) -> (s? t:f=w634:errorcluster)
          }
        }
      }
      frame "Fall Slew Rate" {
        n175 = property class="ChromaAcLoad.lvclass"(reference=w653, error in=w648) -> (reference out=w651:refnum<class "ChromaAcLoad.lvclass">, error out=w650:errorcluster, "Accessors:Device Properties"=w652:T2)
        n176 = for {
          tunnel: w652 -> [w655] mode=indexing
          shift-right: [w656] -> w649
          shift-left: w650 -> [w657]
          stop <- w656 stop-if-true
          n177 = Unbundle By Name(w655) -> ("Phases"=w654:T3)
          n178 = for {
            shift-right: [w663] -> w656
            shift-left: w657 -> [w664]
            tunnel: w654 -> [w662] mode=indexing
            stop <- w663 stop-if-true
            w658 = 4
            w659 = 600
            n179 = Unbundle By Name(w662) -> ("Slew Rate.Fall Slew Rate (Units/S)"=w661:i32)
            n180 = In Range and Coerce(upper limit=w659, x=w661, lower limit=w658) -> (In Range?=w660:bool)  [unwired: 1 out]
            n181 = xnode "Error Ring"("parameter 0"="Fall Slew Rate", "parameter 1"=w661, "parameter 2"=w658, "parameter 3"=w659) -> ("error out"=w665:errorcluster)
            n182 = Select(t=w664, s=w660, f=w665) -> (s? t:f=w663:errorcluster)
          }
        }
      }
    }
  }
  "error out" <- w3
  "ChromaAcLoad out" <- w4
